vi "Control Panel No Objects.vi"(8 "error in (no error)":errorcluster) -> (0 "error out":errorcluster)   [LabVIEW 2009]
uses:
  Main/Global/Flags.vi
  Main/Global/Misc.vi
  Global/GPIB Numbers.vi
  sr830/SR830.lvlib
panel:
  out "ext?OUT":bool
  in  "ext?":bool caption="External Lock"
  in  "ch2form":T1(ring)
  in  "readcontrol":bool
  in  "ch1form":enum16{"X", "R", "X Noise", "Aux 1", "Aux 2"}(ring)
  in  "reset":bool
  out "frequnit":string
  out "freq":dbl caption="Ref Freq"
  out "ch2format":string
  out "ch1format":string
  out "ch2disp":string caption="Channel 2"
  out "ch1disp":string caption="Channel 1"
  in  "readtime":dbl=500.0 caption="Read Time (ms)"
  in  "activeread":bool caption="Auto-read?"
  in  "autophase":bool
  out "phasedisp":dbl caption="Phase"
  out "on":bool caption="Connected"
  out "sensdisp":T2(ring) caption="Sensitivity"
  out "tcdisp":T3(ring) caption="Time Const."
  in  "sens":T2(ring) caption="Sensitivity"
  in  "tc":T3(ring) caption="Time Const."
  in  "connect":bool
  in  "set":bool
  in  "read":bool
  out "active":bool caption="Active"
  in  "endprgm":bool
  # "Lock-in Detector Front Panel"
  # "**Auto-read is just for the output data."
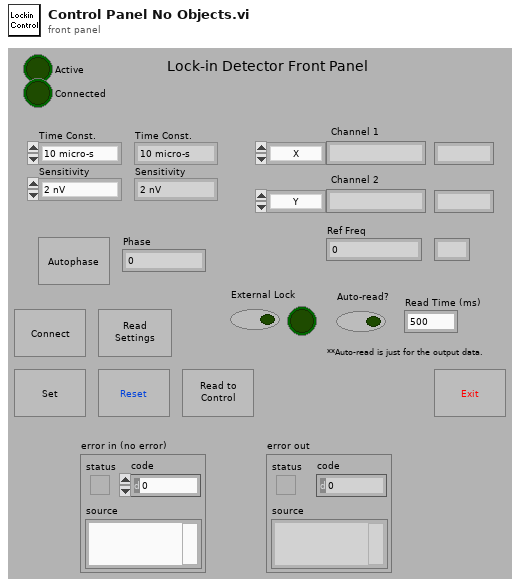
[diagram p1: front panel]
types:
  T1 = enum16{"Y", "Theta", "Y Noise", "Aux 3", "Aux 4"}
  T2 = enum16{"2 nV", "5 nV", "10 nV", "20 nV", "50 nV", "100 nV", "200 nV", "500 nV", "1 microV", "2 microV", "5 microV", "10 microV", "20 microV", "50  microV", "100  microV", "200  microV", "500  microV", "1 mV", "2 mV", "5 mV", "10 mV", "20 mV", "50 mV", "100 mV", "200  mV", "500 mV", "1 V"}
  T3 = enum16{"10 micro-s", "30 micro-s", "100 micro-s", "300 micro-s", "1 ms", "3 ms", "10 ms", "30 ms", "100 ms", "300 ms", "1 s", "3 s", "10 s", "30 s", "100 s", "300 s", "1000 s", "30000 s", "10 ks", "30 ks"}
  T4 = cluster{"name":string, "value":dbl, "unit":string}[]
  T5 = typedef "GPIB Type Def.ctl" = cluster{"Name":string, "bus":dbl, "GPIB":dbl, "GPIB as string":string, "byte":i32, "VISA Resource Name":refnum<visa-resource-name>}
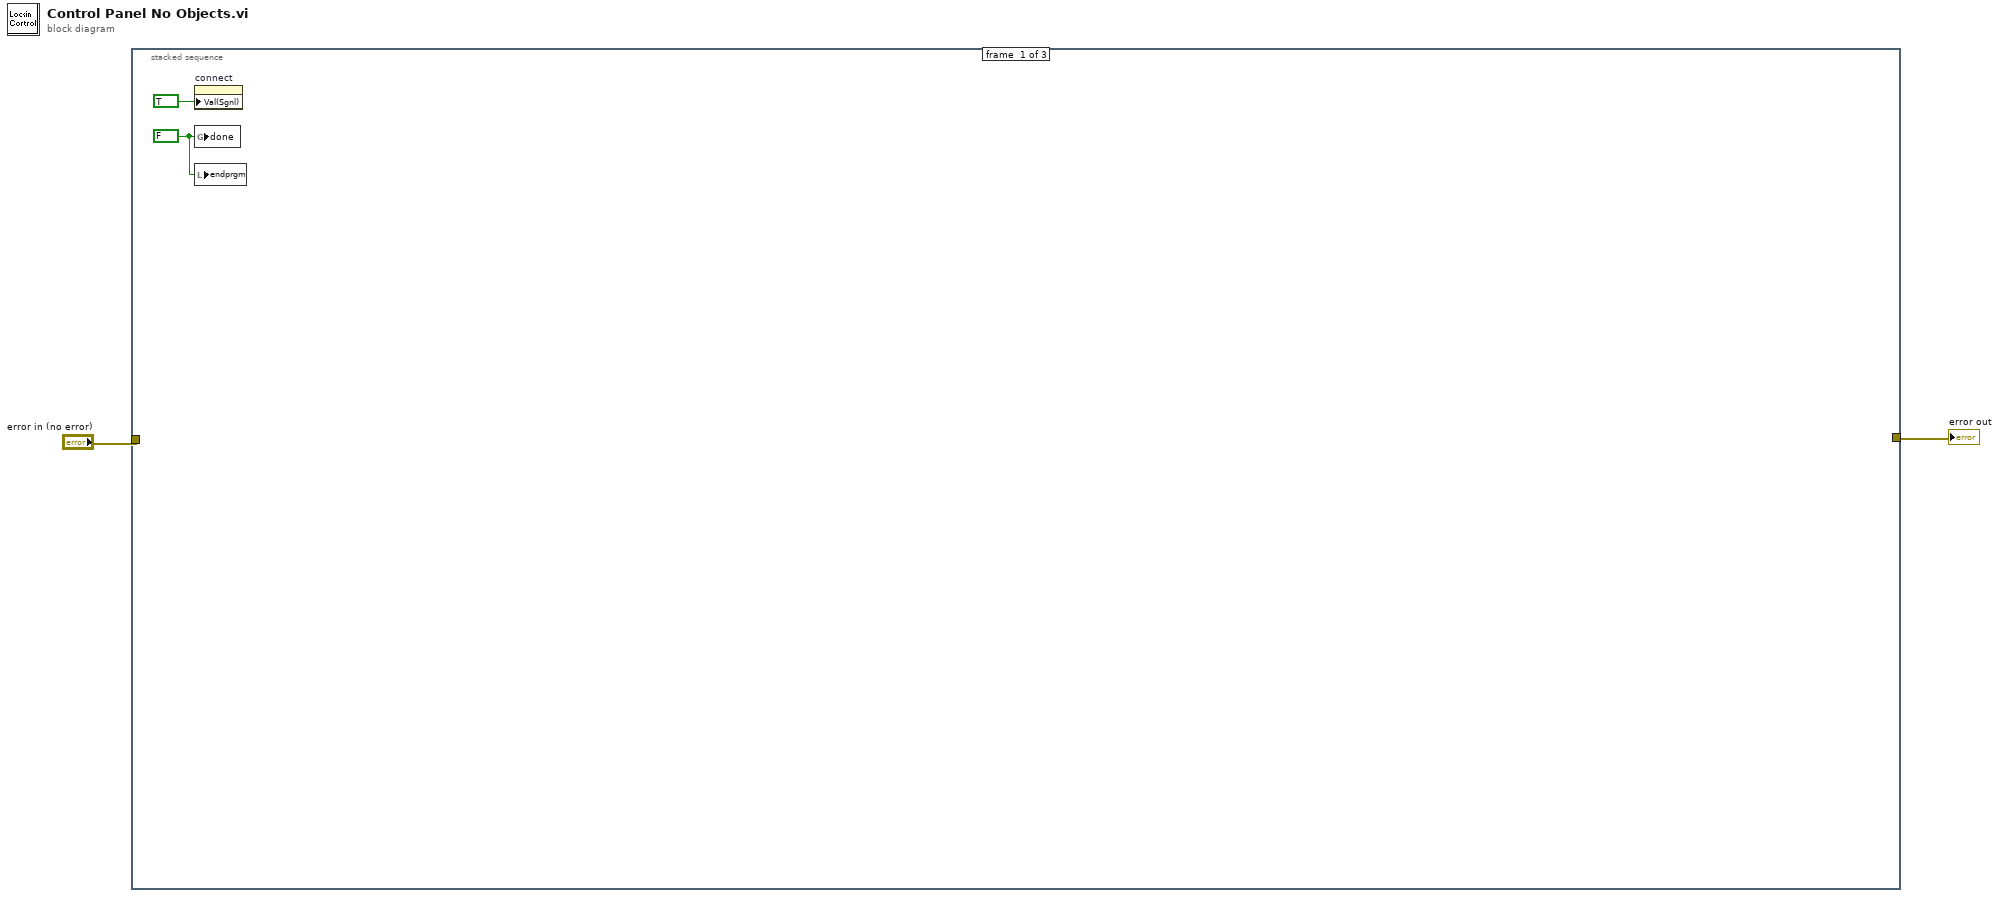
[diagram p0: block diagram]
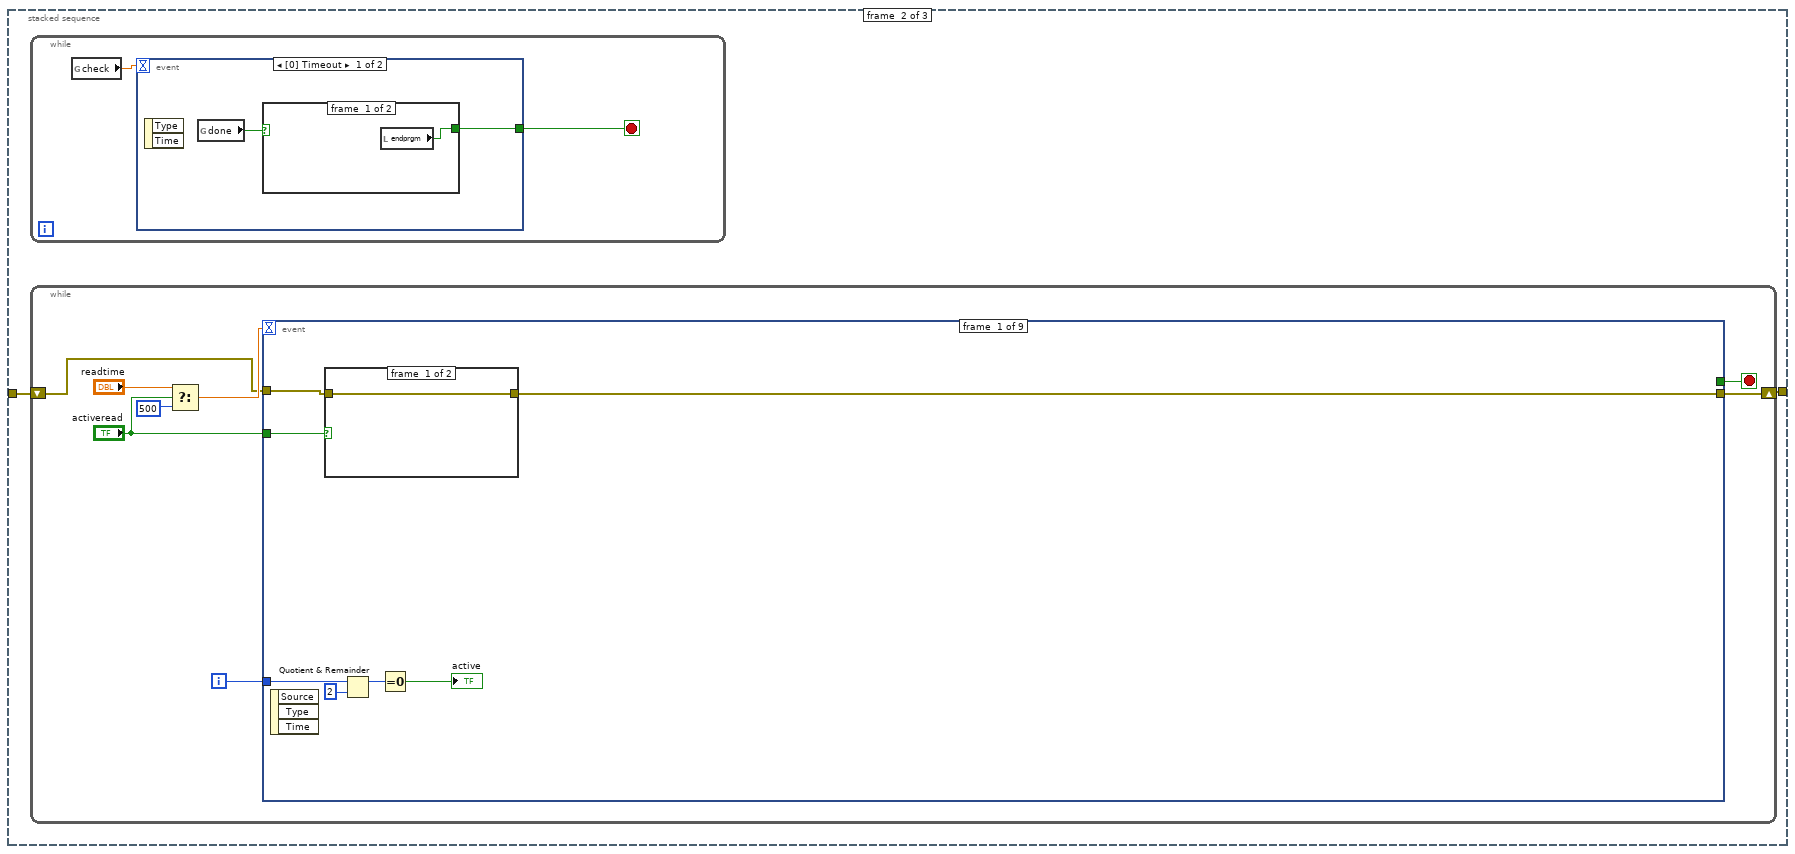
[diagram p2: hidden frame]
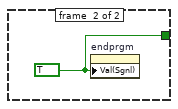
[diagram p3: hidden frame]
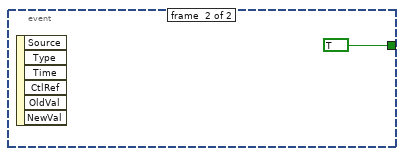
[diagram p4: hidden frame]
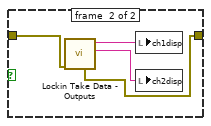
[diagram p5: hidden frame]
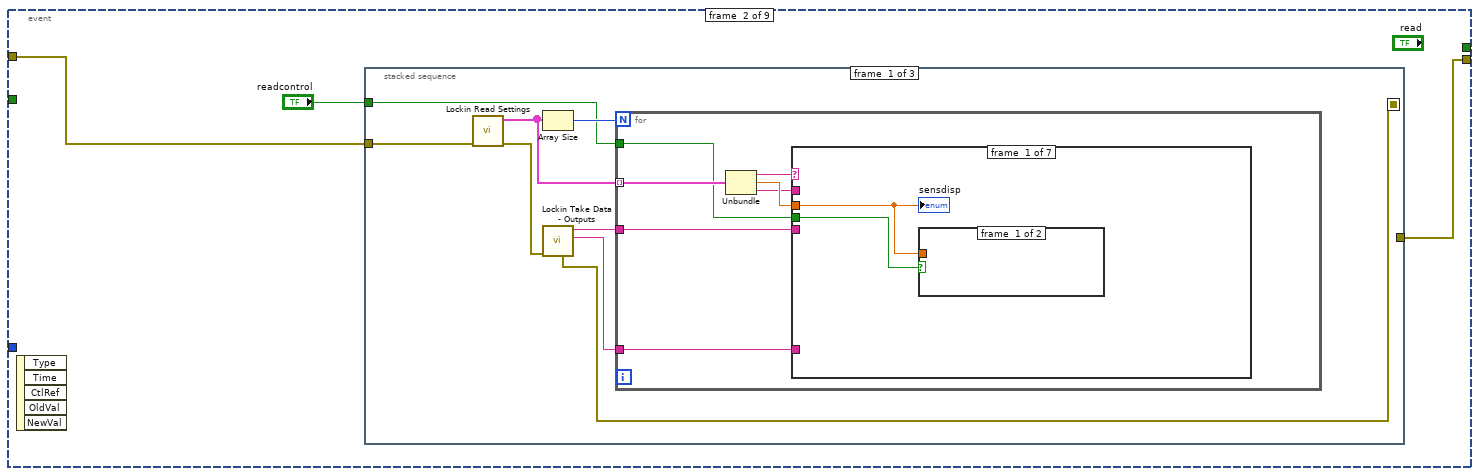
[diagram p6: hidden frame]
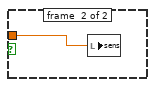
[diagram p7: hidden frame]
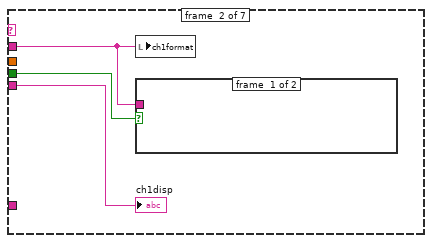
[diagram p8: hidden frame]
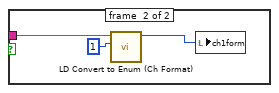
[diagram p9: hidden frame]
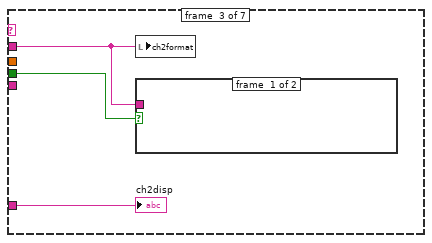
[diagram p10: hidden frame]
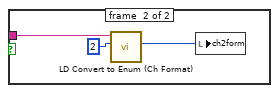
[diagram p11: hidden frame]
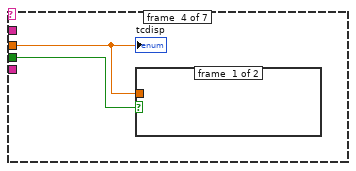
[diagram p12: hidden frame]
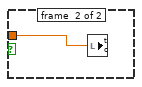
[diagram p13: hidden frame]
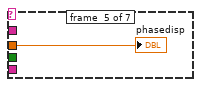
[diagram p14: hidden frame]
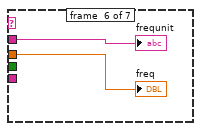
[diagram p15: hidden frame]
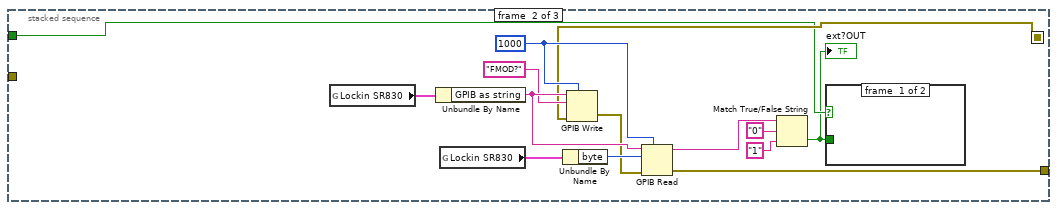
[diagram p17: hidden frame]
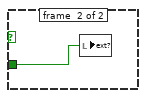
[diagram p18: hidden frame]
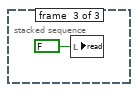
[diagram p19: hidden frame]
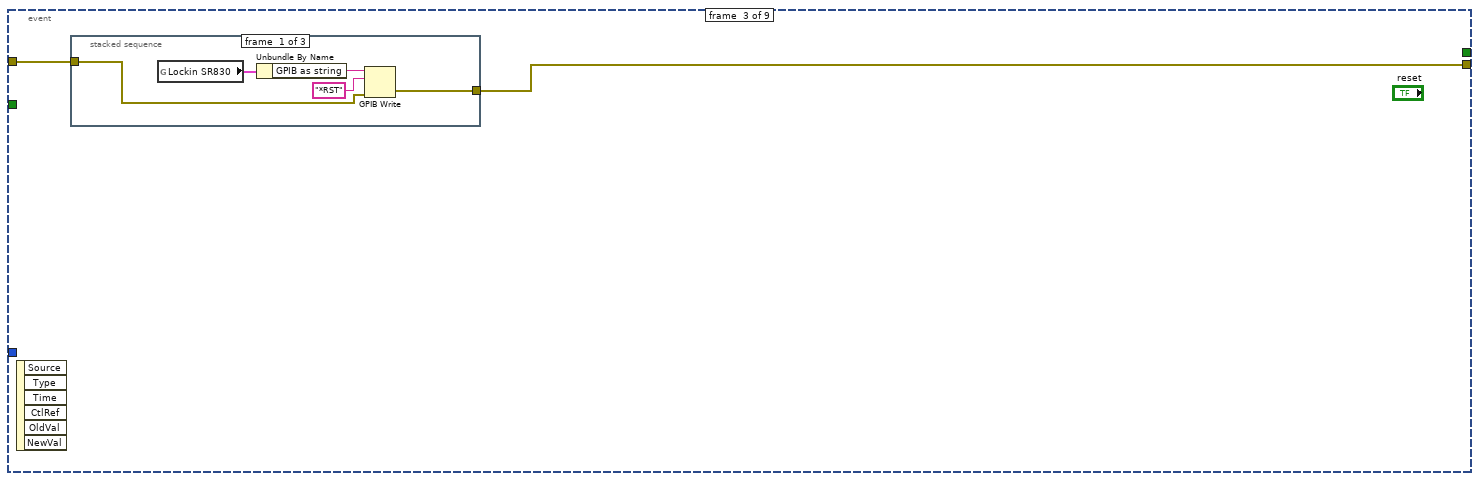
[diagram p20: hidden frame]
diagram:
  n1 = stacked-sequence {
    tunnel: [_ w6 _] -> w2
    tunnel: "error in (no error)" -> [_ w5 _]
    frame #0 {
      w4 = FALSE
      n2 = property on="connect" class="Bool (strict)"("Val(Sgnl)"=TRUE) -> ()  [unwired: 2 in, 2 out]
      n3 = global write "Flags.vi" "done"(w4) -> ()
      n4 = local write "endprgm"(w4) -> ()
    }
    frame #1 {
      n5 = while {
        stop <- w8 stop-if-true
        n6 = global read "Misc.vi" "check"() -> (w7:dbl)
        n7 = event shown="[0] Timeout" {
          selector: _ -> [_ _]
          dyn-events: _ -> [_ _]
          timeout: w7 -> [_ _]
          tunnel: [w9 TRUE] -> w8
          event #0 {
            n8 = event-data() -> ()  [unwired: 3 out]
            n9 = global read "Flags.vi" "done"() -> (w10:bool)
            n10 = case shown="False" w10 {
              tunnel: [w11 w12] -> w9
              frame #0 {
                n11 = local read "endprgm"() -> (w11:bool)
              }
              frame #1 {
                w12 = TRUE
                n12 = property on="endprgm" class="Bool (strict)"("Val(Sgnl)"=w12) -> ()  [unwired: 2 in, 2 out]
              }
            }
          }
          event #1 {
            n13 = event-data() -> ()  [unwired: 7 out]
          }
        }
      }
      n14 = while {
        shift-right: [w15] -> w6
        shift-left: w5 -> [w16]
        i -> [w20]
        stop <- w21 stop-if-true
        n15 = Select(t="readtime", s="activeread", f=500) -> (s? t:f=w17:dbl)
        n16 = event shown="[4] \"set\": Value Change" {
          selector: _ -> [_ _ _ _ _ _ _ _ _]
          dyn-events: _ -> [_ _ _ _ _ _ _ _ _]
          timeout: w17 -> [_ _ _ _ _ _ _ _ _]
          tunnel: [_ _ _ _ _ _ _ _ "endprgm"] -> w21
          tunnel: w20 -> [w25 _ _ _ _ _ _ _ _]
          tunnel: w16 -> [w23 w36 w90 _ w156 w190 w200 w217 w218]
          tunnel: [w22 w35 w89 w97 w155 w186 w199 w217 w218] -> w15
          tunnel: "activeread" -> [w24 _ _ _ _ _ _ _ _]
          event #0 {
            n17 = event-data() -> ()  [unwired: 4 out]
            n18 = case shown="True" w24 {
              tunnel: w23 -> [w29 w33]
              tunnel: [w29 w32] -> w22
              frame #0 {
              }
              frame #1 {
                n19 = call "Lockin Take Data - Outputs.vi"("error in (no error)"=w33) -> ("output2"=w30:string, "output1"=w31:string, "error out"=w32:errorcluster)  [unwired: 8 out]
                n20 = local write "ch1disp"(w31) -> ()
                n21 = local write "ch2disp"(w30) -> ()
              }
            }
            n22 = Quotient & Remainder(x=w25, y=2) -> (x-y*floor(x/y)=w27:i32)  [unwired: 1 out]
            n23 = Equal To 0?(x=w27) -> (x = 0?=→"active":bool)
          }
          event #1 {
            n24 = event-data() -> ()  [unwired: 6 out]
            n25 = stacked-sequence {
              seq-local: [w38 _ _] -> [_ w79 _]
              tunnel: w36 -> [w40 _ _]
              tunnel: [_ w78 _] -> w35
              tunnel: "readcontrol" -> [w37 w74 _]
              frame #0 {
                n26 = call "Lockin Read Settings.vi"("errorIN"=w40) -> ("errorOUT"=w39:errorcluster, "lockinsettings"=w43:T4)  [unwired: 9 out]
                n27 = Array Size(array=w43) -> (size(s)=w44:i32)
                n28 = call "Lockin Take Data - Outputs.vi"("error in (no error)"=w39) -> ("output2"=w41:string, "output1"=w42:string, "error out"=w38:errorcluster)  [unwired: 8 out]
                n29 = for {
                  N: w44 -> [_]
                  tunnel: w43 -> [w51] mode=indexing
                  tunnel: w42 -> [w49]
                  tunnel: w41 -> [w48]
                  tunnel: w37 -> [w45]
                  n30 = Unbundle(w51) -> ("name"=w50:string, "value"=w47:dbl, "unit"=w46:string)
                  n31 = case shown="\"LDch2disp\"" w50 {
                    tunnel: w49 -> [_ w56 _ _ _ _ _]
                    tunnel: w48 -> [_ _ w63 _ _ _ _]
                    tunnel: w47 -> [w52 _ _ w67 w70 w71 _]
                    tunnel: w46 -> [_ w55 w61 _ _ w72 _]
                    tunnel: w45 -> [w53 w57 w62 w68 _ _ _]
                    frame #0 {
                      n32 = case shown="True" w53 {
                        tunnel: w52 -> [_ w54]
                        frame #0 {
                        }
                        frame #1 {
                          n33 = local write "sens"(w54) -> ()
                        }
                      }
                      "sensdisp" <- w52
                    }
                    frame #1 {
                      n34 = local write "ch1format"(w55) -> ()
                      n35 = case shown="True" w57 {
                        tunnel: w55 -> [_ w60]
                        frame #0 {
                        }
                        frame #1 {
                          n36 = call "LD Convert to Enum (Ch Format).vi"("channel"=1, "stringIN"=w60) -> ("ch1form"=w58:enum16{"X", "R", "X Noise", "Aux 1", "Aux 2"})  [unwired: 9 out]
                          n37 = local write "ch1form"(w58) -> ()
                        }
                      }
                      "ch1disp" <- w56
                    }
                    frame #2 {
                      n38 = local write "ch2format"(w61) -> ()
                      n39 = case shown="True" w62 {
                        tunnel: w61 -> [_ w66]
                        frame #0 {
                        }
                        frame #1 {
                          n40 = call "LD Convert to Enum (Ch Format).vi"("channel"=2, "stringIN"=w66) -> ("ch2form"=w64:T1)  [unwired: 9 out]
                          n41 = local write "ch2form"(w64) -> ()
                        }
                      }
                      "ch2disp" <- w63
                    }
                    frame #3 {
                      n42 = case shown="True" w68 {
                        tunnel: w67 -> [_ w69]
                        frame #0 {
                        }
                        frame #1 {
                          n43 = local write "tc"(w69) -> ()
                        }
                      }
                      "tcdisp" <- w67
                    }
                    frame #4 {
                      "phasedisp" <- w70
                    }
                    frame #5 {
                      "freq" <- w71
                      "frequnit" <- w72
                    }
                    frame #6 {
                    }
                  }
                }
              }
              frame #1 {
                w86 = 1000
                n44 = global read "GPIB Numbers.vi" "Lockin SR830"() -> (w81:T5)
                n45 = Unbundle By Name(w81) -> ("GPIB as string"=w85:string)
                n46 = global read "GPIB Numbers.vi" "Lockin SR830"() -> (w83:T5)
                n47 = Unbundle By Name(w83) -> ("byte"=w84:i32)
                n48 = GPIB Write(0:w85, 1:"FMOD?", 3:w79, 4:w86) -> (6:w82:errorcluster)  [unwired: 2 out]
                n49 = GPIB Read(0:w85, 1:w84, 3:w82, 4:w86) -> (5:w77:string, 7:w78:errorcluster)  [unwired: 2 out]
                n50 = Match True/False String(2:"1", 3:"0", 4:w77) -> (0:w73:bool)  [unwired: 1 out]
                "ext?OUT" <- w73
                n51 = case shown="False" w74 {
                  tunnel: w73 -> [_ w87]
                  frame #0 {
                  }
                  frame #1 {
                    n52 = local write "ext?"(w87) -> ()
                  }
                }
              }
              frame #2 {
                n53 = local write "read"(FALSE) -> ()
              }
            }
          }
          event #2 {
            n54 = event-data() -> ()  [unwired: 7 out]
            n55 = stacked-sequence {
              tunnel: w90 -> [w92 _ _]
              tunnel: [w91 _ _] -> w89
              frame #0 {
                n56 = global read "GPIB Numbers.vi" "Lockin SR830"() -> (w95:T5)
                n57 = Unbundle By Name(w95) -> ("GPIB as string"=w94:string)
                n58 = GPIB Write(0:w94, 1:"*RST", 3:w92) -> (6:w91:errorcluster)  [unwired: 3 out]
              }
              frame #1 {
                n59 = Wait (ms)(milliseconds to wait=150) -> ()  [unwired: 1 out]
              }
              frame #2 {
              }
            }
          }
          event #3 {
            n60 = event-data() -> ()  [unwired: 2 out]
            n61 = local write "connect"(FALSE) -> ()
            n62 = call "Lockin Initialize.vi"() -> ("errorOUT"=w98:errorcluster, "ready?"=w100:bool)  [unwired: 1 in, 9 out]
            "on" <- w100
            n63 = case shown="True" w100 {
              tunnel: w98 -> [w101 w114]
              tunnel: [w101 w106] -> w97
              frame #0 {
              }
              frame #1 {
                n64 = call "Lockin Read Settings.vi"("errorIN"=w114) -> ("errorOUT"=w113:errorcluster, "lockinsettings"=w117:T4)  [unwired: 9 out]
                n65 = global read "GPIB Numbers.vi" "Lockin SR830"() -> (w112:T5)
                n66 = call "Lockin Take Data - Outputs.vi"("error in (no error)"=w113) -> ("output2"=w115:string, "output1"=w116:string, "error out"=w107:errorcluster)  [unwired: 8 out]
                n67 = for {
                  tunnel: w117 -> [w123] mode=indexing
                  tunnel: w116 -> [w121]
                  tunnel: w115 -> [w120]
                  n68 = Unbundle(w123) -> ("name"=w122:string, "value"=w119:dbl, "unit"=w118:string)
                  n69 = case shown="\"LDsens\"" w122 {
                    tunnel: w121 -> [_ w126 _ _ _ _ _]
                    tunnel: w120 -> [_ _ w128 _ _ _ _]
                    tunnel: w119 -> [w124 _ _ w129 w130 w131 _]
                    tunnel: w118 -> [_ w125 w127 _ _ w132 _]
                    frame #0 {
                      n70 = local write "sensdisp"(w124) -> ()
                    }
                    frame #1 {
                      n71 = local write "ch1format"(w125) -> ()
                      n72 = local write "ch1disp"(w126) -> ()
                    }
                    frame #2 {
                      n73 = local write "ch2format"(w127) -> ()
                      n74 = local write "ch2disp"(w128) -> ()
                    }
                    frame #3 {
                      n75 = local write "tcdisp"(w129) -> ()
                    }
                    frame #4 {
                      n76 = local write "phasedisp"(w130) -> ()
                    }
                    frame #5 {
                      n77 = local write "freq"(w131) -> ()
                      n78 = local write "frequnit"(w132) -> ()
                    }
                    frame #6 {
                    }
                  }
                }
                n79 = Unbundle By Name(w112) -> ("GPIB as string"=w111:string, "byte"=w108:i32)
                n80 = GPIB Write(0:w111, 1:"FMOD?", 3:w107) -> (6:w109:errorcluster)  [unwired: 3 out]
                n81 = GPIB Read(0:w111, 1:w108, 3:w109) -> (5:w105:string, 7:w106:errorcluster)  [unwired: 3 out]
                n82 = Match True/False String(2:"1", 3:"0", 4:w105) -> (0:w102:bool)  [unwired: 1 out]
                n83 = local write "ext?OUT"(w102) -> ()
              }
            }
          }
          event #4 {
            n84 = event-data() -> ()  [unwired: 7 out]
            n85 = To Long Integer(number="tc") -> (32bit integer=w165:i32)
            n86 = To Long Integer(number="sens") -> (32bit integer=w164:i32)
            n87 = Number To Decimal String(number=w165) -> (decimal integer string=w162:string)  [unwired: 1 out]
            n88 = global read "GPIB Numbers.vi" "Lockin SR830"() -> (w168:T5)
            n89 = Number To Decimal String(number=w164) -> (decimal integer string=w160:string)  [unwired: 1 out]
            n90 = Concatenate Strings("OFLT ", w162) -> (w161:string)
            n91 = Unbundle By Name(w168) -> ("GPIB as string"=w141:string)
            n92 = Number To Decimal String(number="ch1form") -> (decimal integer string=w148:string)  [unwired: 1 out]
            n93 = Concatenate Strings("SENS ", w160) -> (w158:string)
            n94 = local read "ext?"() -> (w135:bool)
            n95 = GPIB Write(0:w141, 1:w161, 3:w156) -> (6:w157:errorcluster)  [unwired: 3 out]
            n96 = Number To Decimal String(number="ch2form") -> (decimal integer string=w146:string)  [unwired: 1 out]
            n97 = Not(x=w135) -> (.not. x?=w134:bool)
            n98 = Concatenate Strings("DDEF 1, ", w148, ",0") -> (w145:string)
            n99 = Boolean To (0,1)(Boolean=w134) -> (0, 1=w133:i16)
            n100 = GPIB Write(0:w141, 1:w158, 3:w157) -> (6:w153:errorcluster)  [unwired: 3 out]
            n101 = Concatenate Strings("DDEF 2, ", w146, ",0") -> (w144:string)
            n102 = GPIB Write(0:w141, 1:w145, 3:w153) -> (6:w152:errorcluster)  [unwired: 3 out]
            n103 = Number To Decimal String(number=w133) -> (decimal integer string=w137:string)  [unwired: 1 out]
            n104 = GPIB Write(0:w141, 1:w144, 3:w152) -> (6:w140:errorcluster)  [unwired: 3 out]
            n105 = Concatenate Strings("FMOD ", w137) -> (w136:string)
            n106 = GPIB Write(0:w141, 1:w136, 3:w140) -> (6:w139:errorcluster)  [unwired: 1 in, 2 out]
            n107 = call "Lockin Read Settings.vi"("errorIN"=w139) -> ("errorOUT"=w155:errorcluster, "lockinsettings"=w154:T4)  [unwired: 9 out]
            n108 = for {
              tunnel: w154 -> [w172] mode=indexing
              n109 = Unbundle(w172) -> ("name"=w171:string, "value"=w170:dbl, "unit"=w169:string)
              n110 = case shown="\"LDfreq\"" w171 {
                tunnel: w170 -> [_ w173 w174 _ _ w178]
                tunnel: w169 -> [_ _ _ w175 w176 w177]
                frame #0 {
                }
                frame #1 {
                  n111 = local write "sensdisp"(w173) -> ()
                }
                frame #2 {
                  n112 = local write "tcdisp"(w174) -> ()
                }
                frame #3 {
                  "ch1format" <- w175
                }
                frame #4 {
                  "ch2format" <- w176
                }
                frame #5 {
                  n113 = local write "freq"(w178) -> ()
                  n114 = local write "frequnit"(w177) -> ()
                }
              }
            }
          }
          event #5 {
            n115 = event-data() -> ()  [unwired: 7 out]
            n116 = Not(x="ext?") -> (.not. x?=w194:bool)
            n117 = Boolean To (0,1)(Boolean=w194) -> (0, 1=w195:i16)
            n118 = global read "GPIB Numbers.vi" "Lockin SR830"() -> (w191:T5)
            n119 = Number To Decimal String(number=w195) -> (decimal integer string=w193:string)  [unwired: 1 out]
            n120 = Unbundle By Name(w191) -> ("byte"=w184:i32, "GPIB as string"=w185:string)
            n121 = Concatenate Strings("FMOD ", w193) -> (w196:string)
            n122 = GPIB Write(0:w185, 1:w196, 3:w190) -> (6:w188:errorcluster)  [unwired: 1 in, 2 out]
            n123 = GPIB Write(0:w185, 1:"FMOD?", 3:w188) -> (6:w187:errorcluster)  [unwired: 1 in, 2 out]
            n124 = GPIB Read(0:w185, 1:w184, 3:w187) -> (5:w181:string, 7:w186:errorcluster)  [unwired: 1 in, 2 out]
            n125 = Match True/False String(2:"1", 3:"0", 4:w181) -> (0:w179:bool)  [unwired: 1 out]
            n126 = local write "ext?OUT"(w179) -> ()
          }
          event #6 {
            n127 = event-data() -> ()  [unwired: 7 out]
            n128 = global read "GPIB Numbers.vi" "Lockin SR830"() -> (w198:T5)
            n129 = Unbundle By Name(w198) -> ("GPIB as string"=w197:string)
            n130 = stacked-sequence {
              seq-local: [w201 _ _] -> [_ _ w206]
              tunnel: w200 -> [w203 _ _]
              tunnel: [_ _ w207] -> w199
              tunnel: w197 -> [w202 _ w215]
              frame #0 {
                n131 = GPIB Write(0:w202, 1:"APHS", 3:w203) -> (6:w201:errorcluster)  [unwired: 3 out]
              }
              frame #1 {
                n132 = Wait (ms)(milliseconds to wait=50) -> ()  [unwired: 1 out]
              }
              frame #2 {
                n133 = global read "GPIB Numbers.vi" "Lockin SR830"() -> (w213:T5)
                n134 = Unbundle By Name(w213) -> ("byte"=w212:i32)
                n135 = GPIB Write(0:w215, 1:"PHAS?", 3:w206) -> (6:w216:errorcluster)  [unwired: 3 out]
                n136 = GPIB Read(0:w215, 1:w212, 2:2, 3:w216) -> (5:w209:string, 7:w210:errorcluster)  [unwired: 2 out]
                n137 = Scan From String(input string=w209, error in=w210) -> (error out=w207:errorcluster, output 1=w208:dbl)  [unwired: 2 in, 3 out]
                n138 = local write "phasedisp"(w208) -> ()
              }
            }
          }
          event #7 {
            n139 = event-data() -> ()  [unwired: 7 out]
          }
          event #8 {
            n140 = event-data() -> ()  [unwired: 7 out]
          }
        }
      }
    }
    frame #2 {
      n141 = local write "endprgm"(FALSE) -> ()
    }
  }
  "error out" <- w2
